vi "uc480_SubVI_Example_GetImageSize.vi"(8 "Error In":errorcluster, 11 ".NET (Reference)":refnum<k24>) -> (0 "Error Out":errorcluster, 1 "Height":i32, 2 "Width":i32, 3 ".NET (Reference)":refnum<k24>)   [LabVIEW 2021]
uses:
  C:/Program Files/Thorlabs/Scientific Imaging/ThorCam/uc480DotNet.dll
panel:
  out "SubSampFacVert":i32
  out "Subsampled Width":i32
  out "Binned Width":i32
  out "Subsampled Height":i32
  out "SubSampFacHor":i32
  out "Factored Width":i32
  out "Factored Height":i32
  out "Binned Height":i32
  out "Scaler":dbl
  out "BinFacVert":i32
  out "BinFaHor":i32
  out "bAbsPosY":bool
  out "bAbsPosX":bool
  out "Max Width":i32
  out "Max Height":i32
  out "s32PosY":i32
  out "s32PosX":i32
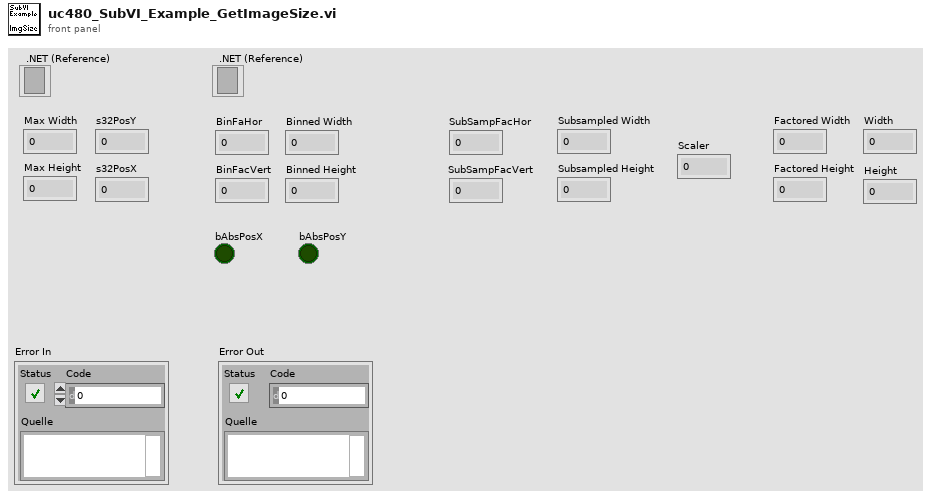
[diagram p1: front panel]
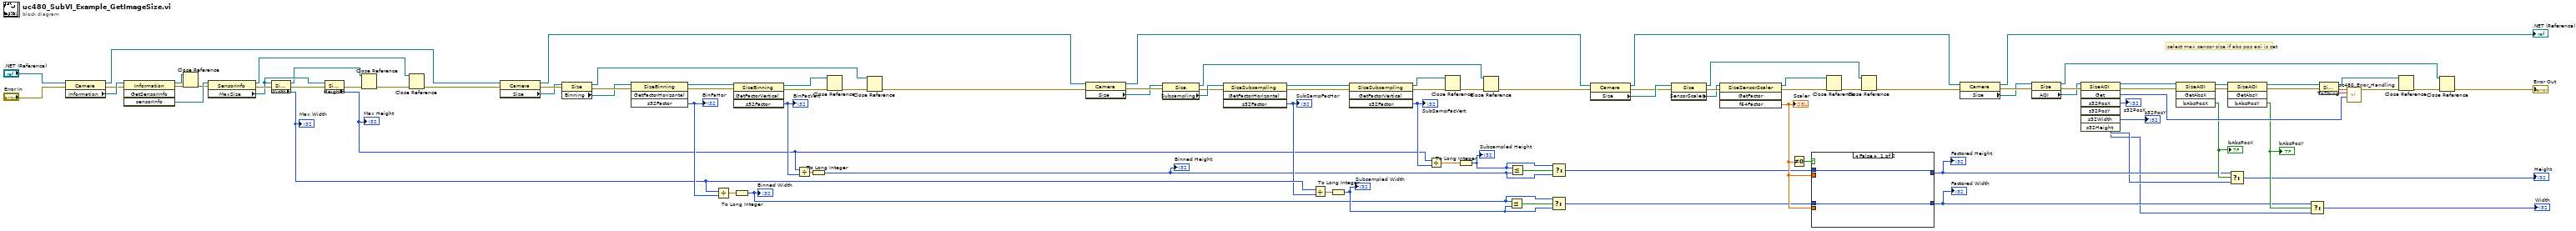
[diagram p0: block diagram]
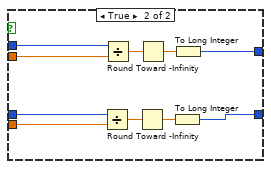
[diagram p2: hidden frame]
diagram:
  # "select max sensor size if abs pos aoi is set"
  n1 = property class="Camera"(reference=".NET (Reference)", error in="Error In") -> (reference out=w34:refnum<k24>, error out=w94:errorcluster, "Information"=w96:refnum<k24>)
  n2 = invoke class="Information" method="GetSensorInfo"(reference=w96, error in=w94) -> (reference out=w37:refnum<k24>, error out=w38:errorcluster, "sensorInfo"=w95:refnum<k24>)  [unwired: 2 in, 1 out]
  n3 = Close Reference(reference=w37, error in (no error)=w38) -> (error out=w39:errorcluster)
  n4 = property class="SensorInfo"(reference=w95, error in=w39) -> (reference out=w35:refnum<k24>, error out=w93:errorcluster, "MaxSize"=w42:refnum<k24>)
  n5 = property class="Size`1[[System.Int32, mscorlib,"(reference=w42, error in=w93) -> (reference out=w41:refnum<k24>, error out=w92:errorcluster, "Width"=w59:i32)
  "Max Width" <- w59
  n6 = property class="Size`1[[System.Int32, mscorlib,"(reference=w42, error in=w92) -> (error out=w40:errorcluster, "Height"=w56:i32)  [unwired: 1 out]
  "Max Height" <- w56
  n7 = Close Reference(reference=w41, error in (no error)=w40) -> (error out=w1:errorcluster)
  n8 = Close Reference(reference=w35, error in (no error)=w1) -> (error out=w36:errorcluster)
  n9 = property on="Eigenschaftsknoten" class="Camera"(reference=w34, error in=w36) -> (reference out=w32:refnum<k24>, error out=w71:errorcluster, "Size"=w47:refnum<k24>)
  n10 = property class="Size"(reference=w47, error in=w71) -> (reference out=w28:refnum<k24>, error out=w80:errorcluster, "Binning"=w79:refnum<k24>)
  n11 = invoke class="SizeBinning" method="GetFactorHorizontal"(reference=w79, error in=w80) -> (reference out=w26:refnum<k24>, error out=w33:errorcluster, "s32Factor"=w60:i32)  [unwired: 2 in, 1 out]
  "BinFaHor" <- w60
  n12 = Divide(x=w59, y=w60) -> (x/y=w63:dbl)
  n13 = invoke class="SizeBinning" method="GetFactorVertical"(reference=w26, error in=w33) -> (reference out=w29:refnum<k24>, error out=w30:errorcluster, "s32Factor"=w61:i32)  [unwired: 2 in, 1 out]
  "BinFacVert" <- w61
  n14 = To Long Integer(number=w63) -> (32bit integer=w50:i32)
  "Binned Width" <- w50
  n15 = Divide(x=w56, y=w61) -> (x/y=w76:dbl)
  n16 = To Long Integer(number=w76) -> (32bit integer=w53:i32)
  "Binned Height" <- w53
  n17 = Close Reference(reference=w29, error in (no error)=w30) -> (error out=w25:errorcluster)
  n18 = Close Reference(reference=w28, error in (no error)=w25) -> (error out=w27:errorcluster)
  n19 = property on="Eigenschaftsknoten" class="Camera"(reference=w32, error in=w27) -> (reference out=w21:refnum<k24>, error out=w31:errorcluster, "Size"=w17:refnum<k24>)
  n20 = property class="Size"(reference=w17, error in=w31) -> (reference out=w16:refnum<k24>, error out=w67:errorcluster, "Subsampling"=w70:refnum<k24>)
  n21 = invoke class="SizeSubsampling" method="GetFactorHorizontal"(reference=w70, error in=w67) -> (reference out=w68:refnum<k24>, error out=w69:errorcluster, "s32Factor"=w57:i32)  [unwired: 2 in, 1 out]
  "SubSampFacHor" <- w57
  n22 = Divide(x=w59, y=w57) -> (x/y=w62:dbl)
  n23 = To Long Integer(number=w62) -> (32bit integer=w51:i32)
  "Subsampled Width" <- w51
  n24 = invoke class="SizeSubsampling" method="GetFactorVertical"(reference=w68, error in=w69) -> (reference out=w23:refnum<k24>, error out=w24:errorcluster, "s32Factor"=w58:i32)  [unwired: 2 in, 1 out]
  "SubSampFacVert" <- w58
  n25 = Divide(x=w56, y=w58) -> (x/y=w66:dbl)
  n26 = Close Reference(reference=w23, error in (no error)=w24) -> (error out=w19:errorcluster)
  n27 = To Long Integer(number=w66) -> (32bit integer=w54:i32)
  "Subsampled Height" <- w54
  n28 = Close Reference(reference=w16, error in (no error)=w19) -> (error out=w18:errorcluster)
  n29 = Less Or Equal?(x=w50, y=w51) -> (x <= y?=w52:bool)
  n30 = Less Or Equal?(x=w54, y=w53) -> (x <= y?=w55:bool)
  n31 = Select(t=w50, s=w52, f=w51) -> (s? t:f=w48:i32)
  n32 = Select(t=w54, s=w55, f=w53) -> (s? t:f=w49:i32)
  n33 = property on="Eigenschaftsknoten" class="Camera"(reference=w21, error in=w18) -> (reference out=w13:refnum<k24>, error out=w20:errorcluster, "Size"=w22:refnum<k24>)
  n34 = property class="Size"(reference=w22, error in=w20) -> (reference out=w8:refnum<k24>, error out=w78:errorcluster, "SensorScaler"=w77:refnum<k24>)
  n35 = invoke class="SizeSensorScaler" method="GetFactor"(reference=w77, error in=w78) -> (reference out=w10:refnum<k24>, error out=w11:errorcluster, "f64Factor"=w65:dbl)  [unwired: 2 in, 1 out]
  "Scaler" <- w65
  n36 = Not Equal To 0?(x=w65) -> (x != 0?=w64:bool)
  n37 = case shown="False" w64 {
    tunnel: w49 -> [w102 w106]
    tunnel: w48 -> [w101 w104]
    tunnel: w65 -> [_ w105]
    tunnel: w65 -> [_ w103]
    tunnel: [w102 w108] -> w74
    tunnel: [w101 w107] -> w73
    frame False {
    }
    frame True {
      n38 = Divide(x=w104, y=w103) -> (x/y=w109:dbl)
      n39 = Divide(x=w106, y=w105) -> (x/y=w112:dbl)
      n40 = Round Toward -Infinity(1:w109) -> (0:w110:dbl)
      n41 = Round Toward -Infinity(1:w112) -> (0:w111:dbl)
      n42 = To Long Integer(number=w110) -> (32bit integer=w107:i32)
      n43 = To Long Integer(number=w111) -> (32bit integer=w108:i32)
    }
  }
  "Factored Height" <- w74
  "Factored Width" <- w73
  n44 = Close Reference(reference=w10, error in (no error)=w11) -> (error out=w9:errorcluster)
  n45 = Close Reference(reference=w8, error in (no error)=w9) -> (error out=w7:errorcluster)
  n46 = property on="Eigenschaftsknoten" class="Camera"(reference=w13, error in=w7) -> (reference out=→".NET (Reference)":refnum<k24>, error out=w15:errorcluster, "Size"=w14:refnum<k24>)
  n47 = property class="Size"(reference=w14, error in=w15) -> (reference out=w3:refnum<k24>, error out=w82:errorcluster, "AOI"=w81:refnum<k24>)
  n48 = invoke class="SizeAOI" method="Get"(reference=w81, error in=w82) -> (reference out=w91:refnum<k24>, error out=w88:errorcluster, "Get"=w85:i32, "s32PosX"=→"s32PosX":i32, "s32PosY"=→"s32PosY":i32, "s32Width"=w43:i32, "s32Height"=w44:i32)  [unwired: 5 in]
  n49 = invoke class="SizeAOI" method="GetAbsX"(reference=w91, error in=w88) -> (reference out=w90:refnum<k24>, error out=w89:errorcluster, "bAbsPosX"=w84:bool)  [unwired: 2 in, 1 out]
  "bAbsPosX" <- w84
  n50 = invoke class="SizeAOI" method="GetAbsY"(reference=w90, error in=w89) -> (reference out=w87:refnum<k24>, error out=w86:errorcluster, "bAbsPosY"=w83:bool)  [unwired: 2 in, 1 out]
  "bAbsPosY" <- w83
  n51 = Select(t=w74, s=w84, f=w44) -> (s? t:f=→"Height":i32)
  n52 = Select(t=w73, s=w83, f=w43) -> (s? t:f=→"Width":i32)
  n53 = invoke class="SizeAOI" method="ToString"(reference=w87, error in=w86) -> (reference out=w5:refnum<k24>, error out=w99:errorcluster, "ToString"=w100:string)  [unwired: 1 in]
  n54 = call "uc480_Error_Handling.vi"("Error Code"=w85, "Error String"=w100, "Error In"=w99) -> ("Error Out"=w6:errorcluster)  [unwired: 8 in]
  n55 = Close Reference(reference=w5, error in (no error)=w6) -> (error out=w4:errorcluster)
  n56 = Close Reference(reference=w3, error in (no error)=w4) -> (error out=→"Error Out":errorcluster)
